vi "Autonomous.vi"() -> ()   [LabVIEW 2017]
doc: "This VI starts when autonomous period begins, and will automatically be terminated when it ends. You can carry out timed or sensor driven operations directly to I/O or to subsystems without needing to return to the caller."
uses:
  Support Code/Routines.ctl
  Support Code/Starting Position.ctl
  <vilib>/Rock Robotics/Network Tables/NT Read String.vi
panel:
  in  "Starting Position":T1
  in  "Routines":T2
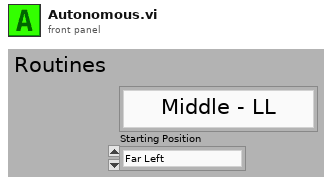
[diagram p1: front panel]
types:
  T1 = typedef "Starting Position.ctl" = enum16{"Far Left", "Middle", "Far Right"}
  T2 = typedef "Routines.ctl" = enum16{"Middle - LL", "Middle - LR", "Middle - RL", "Middle - RR", "Far Right - LL", "Far Right - LR", "Far Right - RL", "Far Right - RR", "Far Left - LL", "Far Left - LR", "Far Left - RL", "Far Left - RR"}
  T3 = typedef "Command Status Info.ctl" = cluster{"Name":string, "Status":T4, "notifier out":T5}
  T4 = typedef "Completion Status.ctl" = enum16{"Successful", "Aborted", "Incomplete"}
  T5 = typedef "Completion Notifier.ctl" = refnum<notifier>
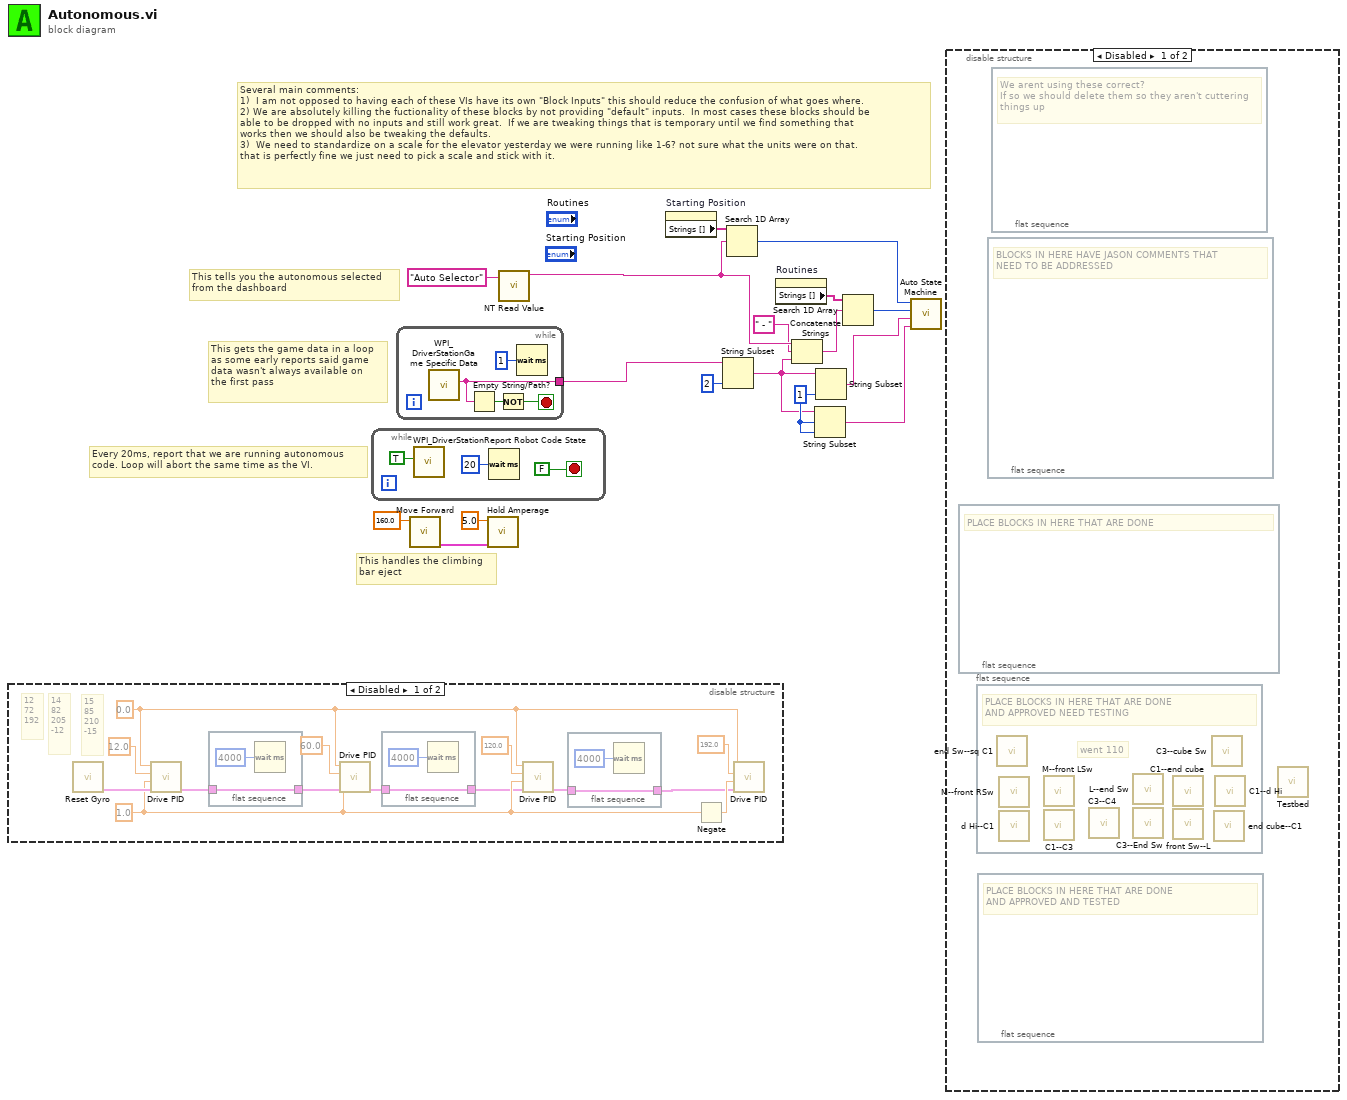
[diagram p0: block diagram]
diagram:
  w7 = 1 ("length (rest)")
  # "This handles the climbing\nbar eject"
  # "This gets the game data in a loop\nas some early reports said game\ndata wasn't always available on\nthe first pass"
  # "Several main comments:\n1)  I am not opposed to having each of these VIs have its own \"Block Inputs\" this should reduce the confusion of what goes where.\n2) We are absolutely killing the fuctionality of these blocks by not providing \"default\" inputs.  In most cases these blocks should be \nable to be dropped with no inputs and still work great.  If we are tweaking things that is temporary until we find something that \nworks then we should also be tweaking the defaults.\n3)  We need to standardize on a scale for the elevator yesterday we were running like 1-6? not sure what the units were on that.\nthat is perfectly fine we just need to pick a scale and stick with it."
  # "This tells you the autonomous selected\nfrom the dashboard"
  # "Every 20ms, report that we are running autonomous\ncode. Loop will abort the same time as the VI."
  n1 = disable-structure shown="Disabled" {
    frame Disabled {
      w29 = 1.0 ("Speed")
      w30 = 0.0 ("Target Angle")
      # "12\n72\n192"
      # "15\n85\n210\n-15"
      # "14\n82\n205\n-12"
      n2 = call "Reset Gyro.vi"() -> ("Command Info Out"=w31:T3)  [unwired: 11 in]
      n3 = call "Drive PID.vi"("Command Info In"=w31, "Speed"=w29, "Distance"=12.0, "Target Angle"=w30) -> ("Command Info Out"=w23:T3)  [unwired: 7 in]
      n4 = flat-sequence {
        tunnel: w23 -> [w36]
        tunnel: [w36] -> w22
        frame #0 {
          n5 = Wait (ms)(milliseconds to wait=u32 4000) -> ()  [unwired: 1 out]
        }
      }
      n6 = call "Drive PID.vi"("Command Info In"=w22, "Speed"=w29, "Distance"=60.0, "Target Angle"=w30) -> ("Command Info Out"=w21:T3)  [unwired: 7 in]
      n7 = flat-sequence {
        tunnel: w21 -> [w34]
        tunnel: [w34] -> w20
        frame #0 {
          n8 = Wait (ms)(milliseconds to wait=u32 4000) -> ()  [unwired: 1 out]
        }
      }
      n9 = call "Drive PID.vi"("Command Info In"=w20, "Speed"=w29, "Distance"=120.0, "Target Angle"=w30) -> ("Command Info Out"=w19:T3)  [unwired: 7 in]
      n10 = flat-sequence {
        tunnel: w19 -> [w32]
        tunnel: [w32] -> w18
        frame #0 {
          n11 = Wait (ms)(milliseconds to wait=u32 4000) -> ()  [unwired: 1 out]
        }
      }
      n12 = Negate(x=w29) -> (-x=w28:dbl)
      n13 = call "Drive PID.vi"("Command Info In"=w18, "Speed"=w28, "Distance"=192.0, "Target Angle"=w30) -> ()  [unwired: 7 in, 1 out]
    }
    frame Enabled {
    }
  }
  n14 = while {
    stop <- FALSE stop-if-true
    n15 = call <vilib>:"WPI_DriverStationReport Robot Code State.vi"("Autonomous"=TRUE) -> ()  [unwired: 10 in, 1 out]
    n16 = Wait (ms)(milliseconds to wait=u32 20) -> ()  [unwired: 1 out]
  }
  n17 = while {
    tunnel: [w43] -> w16
    stop <- w42 stop-if-true
    n18 = call <vilib>:"WPI_DriverStationGame Specific Data.vi"() -> ("Game Specific Data"=w43:string)  [unwired: 11 in]
    n19 = Empty String/Path?(string/path=w43) -> (empty?=w44:bool)
    n20 = Not(x=w44) -> (.not. x?=w42:bool)
    n21 = Wait (ms)(milliseconds to wait=u32 1) -> ()  [unwired: 1 out]
  }
  n22 = call "Move Forward.vi"("Setpoint"=160.0) -> ("Command Info Out"=w14:T3)  [unwired: 10 in]
  n23 = call "Hold Amperage.vi"("Command Info In"=w14, "Setpoint"=5.0) -> ()  [unwired: 9 in, 1 out]
  n24 = call-poly <vilib>:"NT Read Value.vi"("Name"="Auto Selector") -> ("String"=w12:string)  [unwired: 9 in, 1 out]
  n25 = property on="Starting Position" class="Enum (strict)"() -> ("Strings []"=w1:string[])  [unwired: 2 in, 2 out]
  n26 = String Subset(string=w16, length (rest)=2 ("length (rest)")) -> (substring=w4:string)  [unwired: 1 in]
  n27 = Search 1D Array(1D array=w1, element=w12) -> (index of element=w9:i32)  [unwired: 1 in]
  n28 = property on="Routines" class="Enum (strict)"() -> ("Strings []"=w2:string[])  [unwired: 2 in, 2 out]
  n29 = Concatenate Strings(w12, " - " ("string"), w4) -> (w8:string)
  n30 = String Subset(string=w4, offset (0)=w7, length (rest)=w7) -> (substring=w5:string)
  n31 = String Subset(string=w4, length (rest)=w7) -> (substring=w6:string)  [unwired: 1 in]
  n32 = Search 1D Array(1D array=w2, element=w8) -> (index of element=w10:i32)  [unwired: 1 in]
  n33 = call "Auto State Machine.vi"("Scale"=w5, "Switch"=w6, "index of element"=w10, "Starting Position"=w9) -> ()  [unwired: 8 in]
  n34 = disable-structure shown="Disabled" {
    frame Disabled {
      n35 = flat-sequence {
        frame #0 {
          # "PLACE BLOCKS IN HERE THAT ARE DONE"
        }
      }
      n36 = flat-sequence {
        frame #0 {
          # "went 110"
          # "PLACE BLOCKS IN HERE THAT ARE DONE\nAND APPROVED NEED TESTING"
          n37 = call "end Sw--sq C1.vi"() -> ()  [unwired: 11 in, 1 out]
          n38 = call "M--front RSw.vi"() -> ()  [unwired: 11 in, 1 out]
          n39 = call "d Hi--C1.vi"() -> ()  [unwired: 11 in, 1 out]
          n40 = call "M--front LSw.vi"() -> ()  [unwired: 11 in, 1 out]
          n41 = call "C1--C3.vi"() -> ()  [unwired: 10 in, 1 out]
          n42 = call "C3--C4.vi"() -> ()  [unwired: 11 in, 1 out]
          n43 = call "L--end Sw.vi"() -> ()  [unwired: 9 in, 1 out]
          n44 = call "C3--End Sw.vi"() -> ()  [unwired: 11 in, 1 out]
          n45 = call "C1--end cube.vi"() -> ()  [unwired: 11 in, 1 out]
          n46 = call "front Sw--L.vi"() -> ()  [unwired: 11 in, 1 out]
          n47 = call "C3--cube Sw.vi"() -> ()  [unwired: 11 in, 1 out]
          n48 = call "end cube--C1.vi"() -> ()  [unwired: 11 in, 1 out]
          n49 = call "C1--d Hi.vi"() -> ()  [unwired: 11 in, 1 out]
        }
      }
      n50 = flat-sequence {
        frame #0 {
          # "PLACE BLOCKS IN HERE THAT ARE DONE\nAND APPROVED AND TESTED"
        }
      }
      n51 = flat-sequence {
        frame #0 {
          # "BLOCKS IN HERE HAVE JASON COMMENTS THAT\nNEED TO BE ADDRESSED"
        }
      }
      n52 = flat-sequence {
        frame #0 {
          # "We arent using these correct?\nIf so we should delete them so they aren't cuttering things up"
        }
      }
      n53 = call "Testbed.vi"() -> ()  [unwired: 12 in]
    }
    frame Enabled {
    }
  }
